vi "ErrorViewer.CreateRequests.vi"(8 "error in (no error)":errorcluster) -> (0 "error out":errorcluster, 3 "Requests":T1)   [LabVIEW 2024, in "ErrorViewer.lvclass"]
uses:
  ErrorViewer.lvclass
  ErrorViewer.lvclass/ErrorViewer.ctl
  Request Events--cluster.ctl
  Do Something Args.ctl
  RQMHCore/ModuleCore/Reply.ctl
  RQMHCore/ModuleCore/Module.lvclass
  InjectLogEvent.ctl
  RQMHCore/ErrorReporting/Record/LogRecord.lvclass
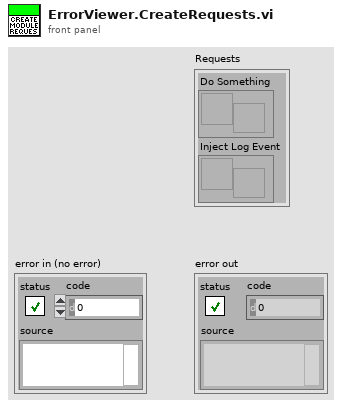
[diagram p1: front panel]
types:
  T1 = typedef "ErrorViewer.lvclass/Request Events--cluster.ctl" = cluster{"Do Something":refnum<user-event>, "Inject Log Event":refnum<user-event>}
  T2 = typedef "ErrorViewer.lvclass/InjectLogEvent.ctl" = cluster{"Log Event":refnum<user-event>}
  T3 = typedef "Module.lvclass/Reply.ctl" = cluster{"Expects Reply":bool, "Reply":refnum<notifier>}
  T4 = typedef "ErrorViewer.lvclass/Do Something Args.ctl" = cluster{"Msg":string}
  T5 = cluster{"Do Something Args":T4, "Reply Payload":T3}
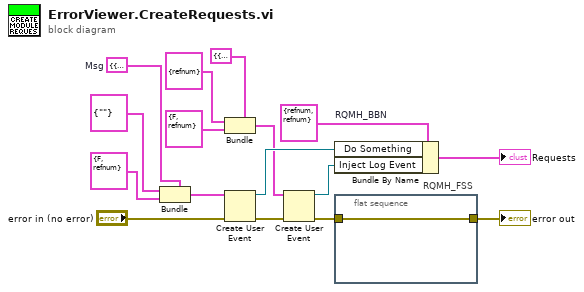
[diagram p0: block diagram]
diagram:
  w10 = T5 {"Do Something Args"={"Msg"=""}, "Reply Payload"={"Expects Reply"=FALSE, "Reply"=refnum}}  # Msg
  n1 = Bundle(cluster=w10, "Do Something Args"=T4 {"Msg"=""}, "Reply Payload"=T3 {"Expects Reply"=FALSE, "Reply"=refnum}) -> (w13:T5)
  n2 = Bundle(cluster=cluster{"Args":T2, "Reply Payload":T3} {"Args"={"Log Event"=refnum}, "Reply Payload"={"Expects Reply"=FALSE, "Reply"=refnum}}, "Args"=T2 {"Log Event"=refnum}, "Reply Payload"=T3 {"Expects Reply"=FALSE, "Reply"=refnum}) -> (w6:cluster{"Args":T2, "Reply Payload":T3})
  n3 = Create User Event(user event datatype=w13, error in="error in (no error)") -> (user event=w9:refnum<user-event>, error out=w4:errorcluster)
  n4 = Create User Event(user event datatype=w6, error in=w4) -> (user event=w1:refnum<user-event>, error out=w3:errorcluster)
  n5 = Bundle By Name "RQMH_BBN"(cluster=T1 {"Do Something"=refnum, "Inject Log Event"=refnum} ("Requests"), "Do Something"=w9, "Inject Log Event"=w1) -> (→"Requests":T1)
  n6 = flat-sequence "RQMH_FSS" {
    tunnel: [w17] -> w8
    tunnel: w3 -> [w17]
    frame #0 {
    }
  }
  "error out" <- w8
